vi "5_Solve_Data_SubVI.vi"(11 "String":string) -> (1 "Phase Data":dbl, 2 "Frequency Data (Hz)":dbl, 3 "Enum":T1(ring))   [LabVIEW 2024]
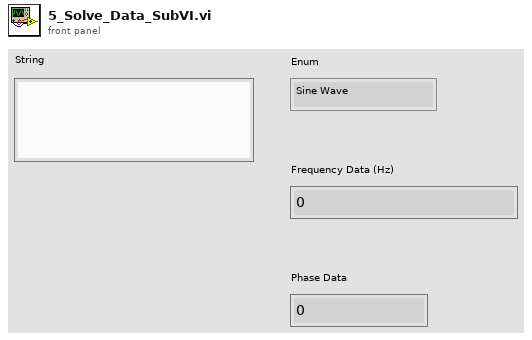
[diagram p1: front panel]
types:
  T1 = enum16{"Sine Wave", "Triangular Wave", "Square Wave"}
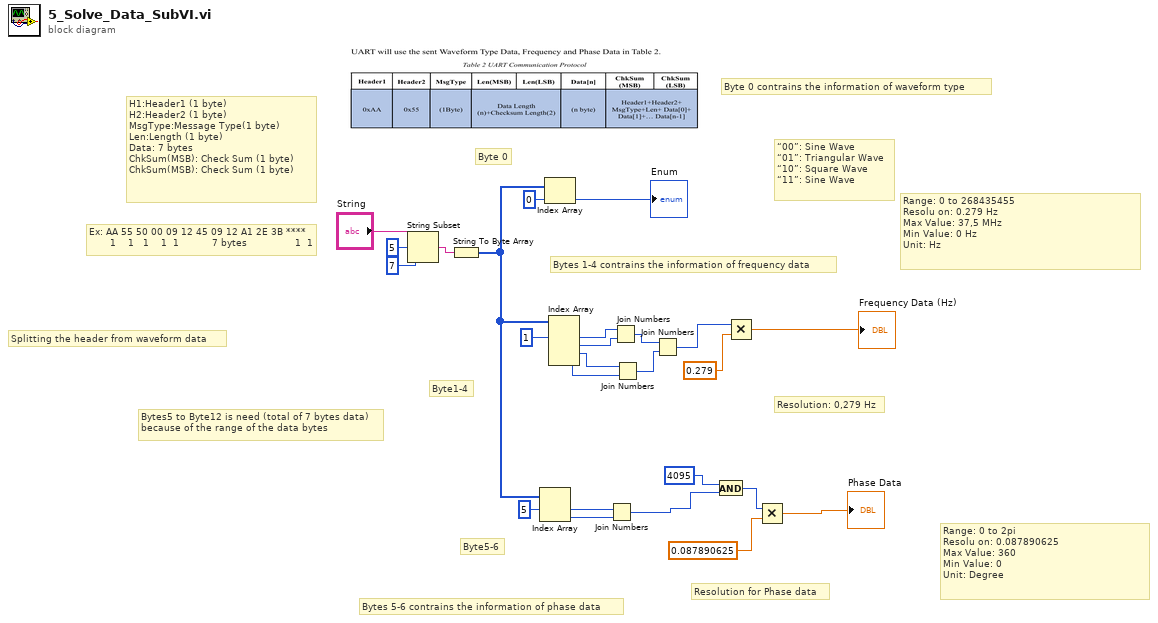
[diagram p0: block diagram]
diagram:
  # "Bytes 5-6 contrains the information of phase data"
  # "Bytes 1-4 contrains the information of frequency data"
  # "Byte 0 contrains the information of waveform type"
  # "Splitting the header from waveform data"
  # "Range: 0 to 2pi                                    \nResolu on: 0.087890625 \nMax Value: 360                                          \nMin Value: 0  \nUnit: Degree"
  # "Range: 0 to 268435455 \nResolu on: 0.279 Hz                                          \nMax Value: 37,5 MHz                                          \nMin Value: 0 Hz \nUnit: Hz"
  # "“00”: Sine Wave \n“01”: Triangular Wave \n“10”: Square Wave \n“11”: Sine Wave"
  # "Bytes5 to Byte12 is need (total of 7 bytes data)\nbecause of the range of the data bytes"
  # "Ex: AA 55 50 00 09 12 45 09 12 A1 2E 3B ****\n       1    1   1    1  1           7 bytes                1  1"
  # "H1:Header1 (1 byte)\nH2:Header2 (1 byte)\nMsgType:Message Type(1 byte)\nLen:Length (1 byte)\nData: 7 bytes\nChkSum(MSB): Check Sum (1 byte)\nChkSum(MSB): Check Sum (1 byte)"
  # "Byte 0"
  # "Byte1-4"
  # "Byte5-6"
  # "Resolution for Phase data"
  # "Resolution: 0,279 Hz"
  n1 = String Subset(string="String", offset (0)=5, length (rest)=7 ("length (rest)")) -> (substring=w6:string)
  n2 = String To Byte Array(string=w6) -> (unsigned byte array=w10:u8[])
  n3 = Index Array(array=w10, index #1=5 ("index")) -> (element #1=w17:u8, element #2=w18:u8)  [unwired: 1 in]
  n4 = Index Array "Index Array"(array=w10, index=0) -> (element=→"Enum":u8)
  n5 = Index Array(array=w10, index #1=1 ("index")) -> (element #1=w13:u8, element #2=w14:u8, element #3=w15:u8, element #4=w16:u8)  [unwired: 3 in]
  n6 = Join Numbers(hi=w17, lo=w18) -> ((hi.lo)=w3:u16)
  n7 = Join Numbers(hi=w13, lo=w14) -> ((hi.lo)=w21:u16)
  n8 = Join Numbers(hi=w15, lo=w16) -> ((hi.lo)=w22:u16)
  n9 = Join Numbers(hi=w21, lo=w22) -> ((hi.lo)=w23:u32)
  n10 = And(x=u16 4095, y=w3) -> (x .and. y?=w1:u16)
  n11 = Multiply(x=w23, y=0.279) -> (x*y=→"Frequency Data (Hz)":dbl)
  n12 = Multiply(x=w1, y=0.087890625) -> (x*y=→"Phase Data":dbl)
